vi "POST.vi"(7 "LabVIEW Web Service Request":refnum<class "Web Request.lvclass">) -> ()   [LabVIEW 2019]
uses:
  <vilib>/wsapi/Web Request.lvclass
panel:
  # "Use the Web Service Request input terminal to call the VIs on the Web Services palette. Do not remove it from the connector pane unless you don't need access to the palette."
  # "Each additional control wired to the connector pane will be available as an input in the URL. To include an indicator in terminal-mode output (the default setting), it must also be wired to the connector pane."
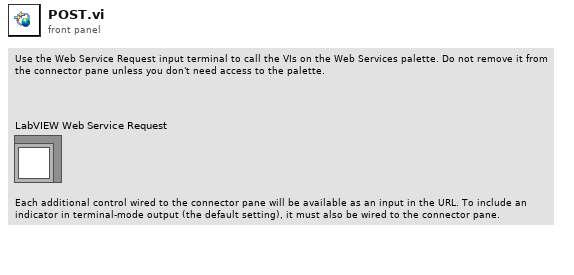
[diagram p1: front panel]
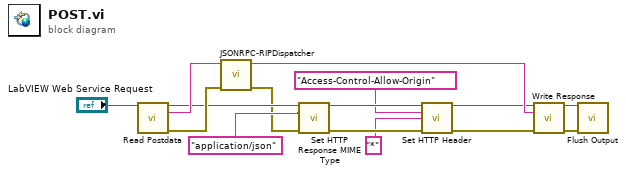
[diagram p0: block diagram]
diagram:
  n1 = call <vilib>:"Read Postdata.vi"("LabVIEW Web Service Request"="LabVIEW Web Service Request") -> ("LabVIEW Web Service Request out"=w9:refnum<class "Web Request.lvclass">, "postdata"=w12:string, "error out"=w13:errorcluster)  [unwired: 12 in]
  n2 = call "JSONRPC-RIPDispatcher.vi"("error in"=w13, "input string"=w12) -> ("error out"=w7:errorcluster, "response"=w11:string)  [unwired: 8 in]
  n3 = call <vilib>:"Set HTTP Response MIME Type.vi"("LabVIEW Web Service Request"=w9, "MIME type (text/html)"="application/json" ("header"), "error in (no error)"=w7) -> ("LabVIEW Web Service Request out"=w6:refnum<class "Web Request.lvclass">, "error out"=w5:errorcluster)  [unwired: 11 in]
  n4 = call <vilib>:"Set HTTP Header.vi"("LabVIEW Web Service Request"=w6, "header"="Access-Control-Allow-Origin", "header value"="*", "error in (no error)"=w5) -> ("LabVIEW Web Service Request out"=w4:refnum<class "Web Request.lvclass">, "error out"=w3:errorcluster)  [unwired: 10 in]
  n5 = call <vilib>:"Write Response.vi"("LabVIEW Web Service Request"=w4, "response string"=w11, "error in (no error)"=w3) -> ("LabVIEW Web Service Request out"=w15:refnum<class "Web Request.lvclass">, "error out"=w14:errorcluster)  [unwired: 11 in]
  n6 = call <vilib>:"Flush Output.vi"("LabVIEW Web Service Request"=w15, "error in (no error)"=w14) -> ()  [unwired: 12 in, 2 out]
